vi "AlarmBuzzer.vi"() -> ()   [LabVIEW 2024]
uses:
  Driver/CTIPicoVISA.lvlib
panel:
  out "Alarm":bool
  out "current time":timestamp
  in  "Time Stamp":timestamp
  in  "Freq Hz":sgl(slide) scale=0.0..20000.0
  in  "Duty % (0-1)":sgl(slide) scale=0.0..1.0
  out "Identity":T1
  in  "GroveConnector":enum16{"A0", "A1", "A2"}(ring)
  in  "stop":bool
  in  "VISA resource name in":refnum<visa-resource-name>="COM7"
  out "error out":errorcluster
  # "https://wiki.seeedstudio.com/Grove-Passive-Buzzer/"
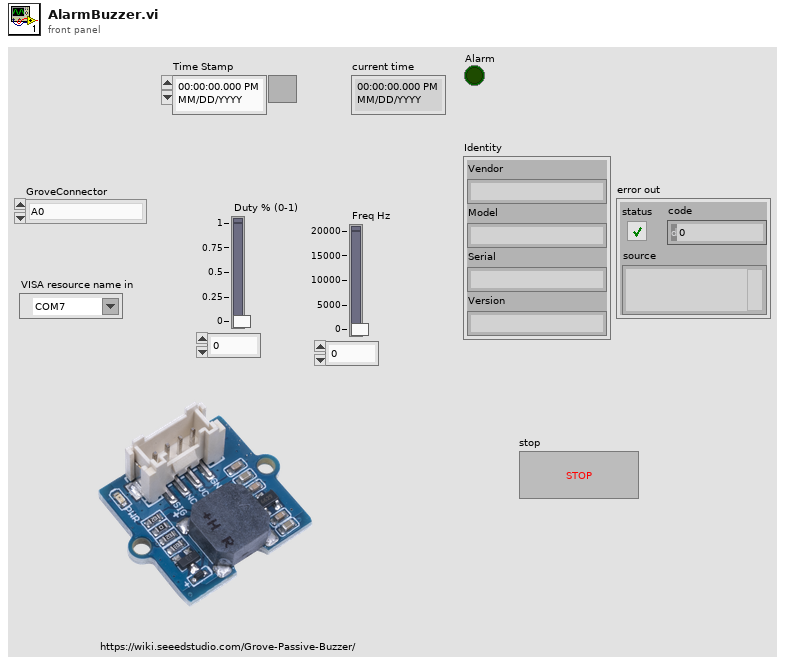
[diagram p1: front panel]
types:
  T1 = cluster{"Vendor":string, "Model":string, "Serial":string, "Version":string}
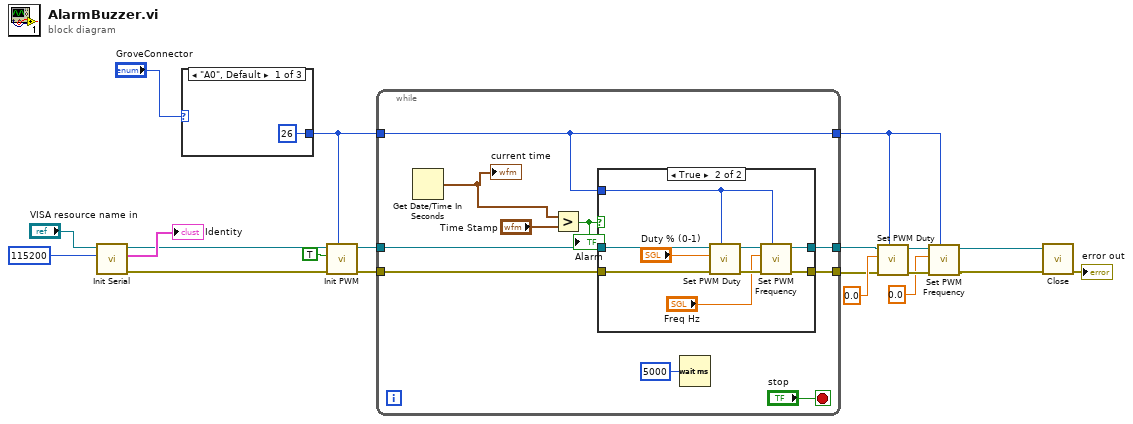
[diagram p0: block diagram]
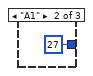
[diagram p2: hidden frame]
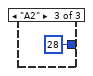
[diagram p3: hidden frame]
diagram:
  n1 = call "Init Serial.vi"("Baud (115200)"=u32 115200, "VISA resource name in"="VISA resource name in") -> ("error out"=w14:errorcluster, "Identity"=→"Identity":T1, "VISA resource name Out"=w15:refnum<visa-resource-name>)  [unwired: 7 in]
  n2 = case shown="\"A0\", Default" "GroveConnector" {
    tunnel: [26 ("GPIO") 27 ("GPIO") 28 ("GPIO")] -> w13
    frame "A0", Default {
    }
    frame "A1" {
    }
    frame "A2" {
    }
  }
  n3 = call "Init PWM.vi"("GPIO"=w13, "error in (no error)"=w14, "Enable (F)"=TRUE, "VISA resource name in"=w15) -> ("error out"=w11:errorcluster, "VISA resource name"=w10:refnum<visa-resource-name>)  [unwired: 6 in]
  n4 = while {
    tunnel: w10 -> [w30]
    tunnel: w13 -> [w27]
    tunnel: w11 -> [w31]
    tunnel: [w29] -> w4
    tunnel: [w28] -> w5
    tunnel: [w27] -> w3
    stop <- "stop" stop-if-true
    n5 = Get Date/Time In Seconds() -> (seconds since 1Jan1904=w24:timestamp)
    "current time" <- w24
    n6 = Greater?(x=w24, y="Time Stamp") -> (0:w26:bool)
    "Alarm" <- w26
    n7 = case shown="True" w26 {
      tunnel: w31 -> [w34 w44]
      tunnel: w30 -> [w35 w42]
      tunnel: [w34 w40] -> w29
      tunnel: [w35 w39] -> w28
      tunnel: w27 -> [_ w38]
      frame False {
      }
      frame True {
        n8 = call "Set PWM Duty.vi"("GPIO"=w38, "error in (no error)"=w44, "Duty % (0-1)"="Duty % (0-1)", "VISA resource name in"=w42) -> ("error out"=w43:errorcluster, "VISA resource name"=w41:refnum<visa-resource-name>)  [unwired: 6 in]
        n9 = call "Set PWM Frequency.vi"("GPIO"=w38, "error in (no error)"=w43, "Freq Hz"="Freq Hz", "VISA resource name in"=w41) -> ("error out"=w40:errorcluster, "VISA resource name"=w39:refnum<visa-resource-name>)  [unwired: 6 in]
      }
    }
    n10 = Wait (ms)(milliseconds to wait=u32 5000) -> ()  [unwired: 1 out]
  }
  n11 = call "Set PWM Duty.vi"("GPIO"=w3, "error in (no error)"=w4, "Duty % (0-1)"=sgl 0.0, "VISA resource name in"=w5) -> ("error out"=w9:errorcluster, "VISA resource name"=w8:refnum<visa-resource-name>)  [unwired: 6 in]
  n12 = call "Set PWM Frequency.vi"("GPIO"=w3, "error in (no error)"=w9, "Freq Hz"=sgl 0.0, "VISA resource name in"=w8) -> ("error out"=w1:errorcluster, "VISA resource name"=w2:refnum<visa-resource-name>)  [unwired: 6 in]
  n13 = call "Close.vi"("error in (no error)"=w1, "VISA resource name in"=w2) -> ("error out"=→"error out":errorcluster)  [unwired: 9 in]
